vi "uc480_GetCameraList.vi"() -> ()   [LabVIEW 2011]
uses:
  C:/Program Files/Thorlabs/Scientific Imaging/DCx Camera Support/Develop/DotNet/uc480DotNet.dll
  Develop/DotNet/uc480DotNet.dll
panel:
  out "Ser.No. Camera 9":string
  out "Ser.No. Camera 8":string
  out "Ser.No. Camera 7":string
  out "Ser.No. Camera 6":string
  out "Ser.No. Camera 5":string
  out "Ser.No. Camera 4":string
  out "Ser.No. Camera 3":string
  out "Ser.No. Camera 2":string
  out "Ser.No. Camera 1":string
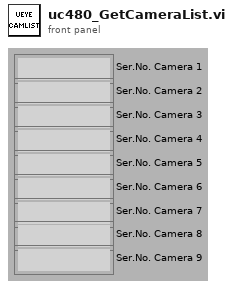
[diagram p1: front panel]
types:
  T1 = cluster{"CameraList[0]":refnum<k24>, "CameraList[1]":refnum<k24>, "CameraList[2]":refnum<k24>, "CameraList[3]":refnum<k24>, "CameraList[4]":refnum<k24>, "CameraList[5]":refnum<k24>, "CameraList[6]":refnum<k24>, "CameraList[7]":refnum<k24>, "CameraList[8]":refnum<k24>}
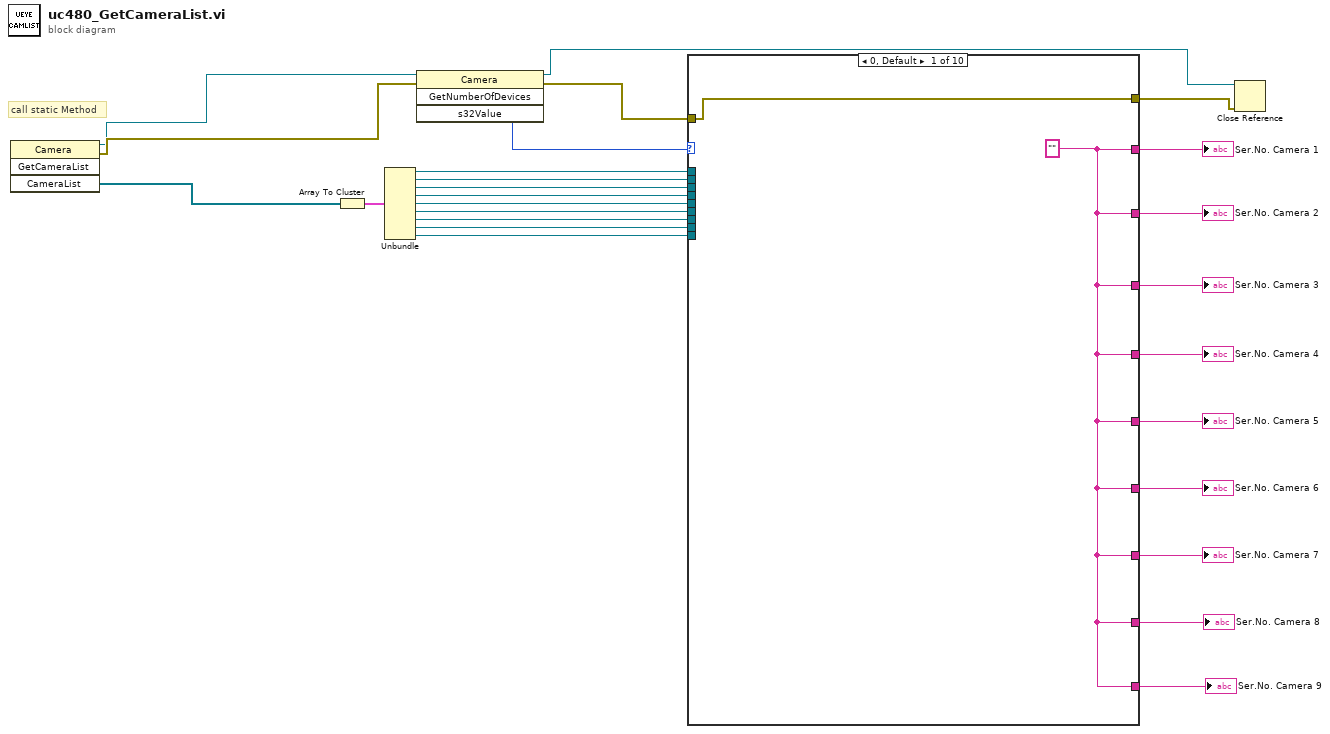
[diagram p0: block diagram]
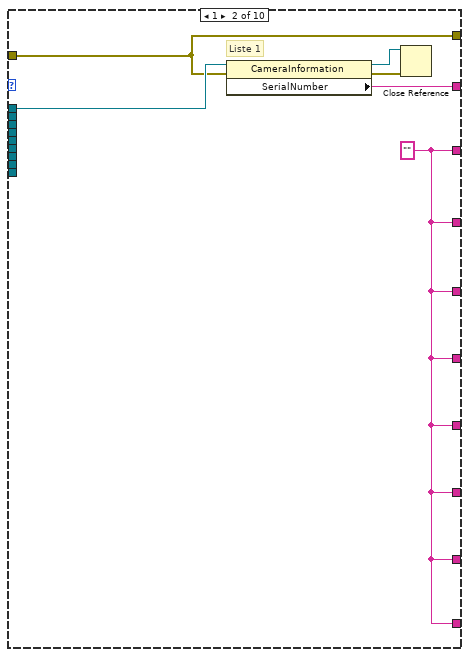
[diagram p2: hidden frame]
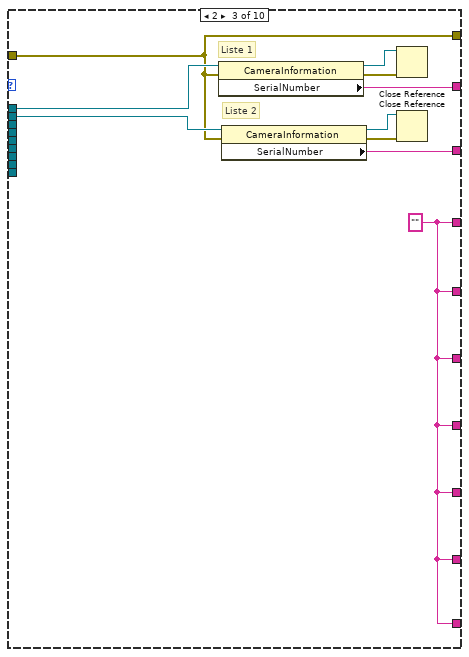
[diagram p3: hidden frame]
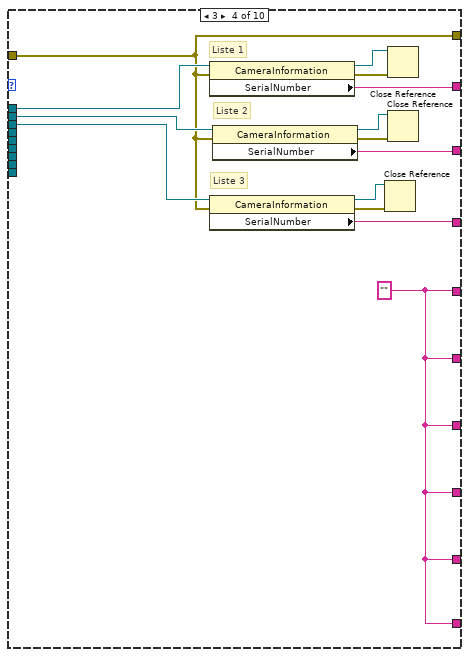
[diagram p4: hidden frame]
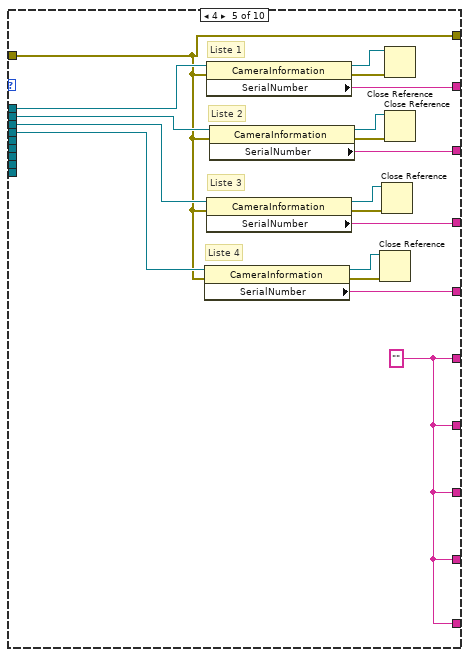
[diagram p5: hidden frame]
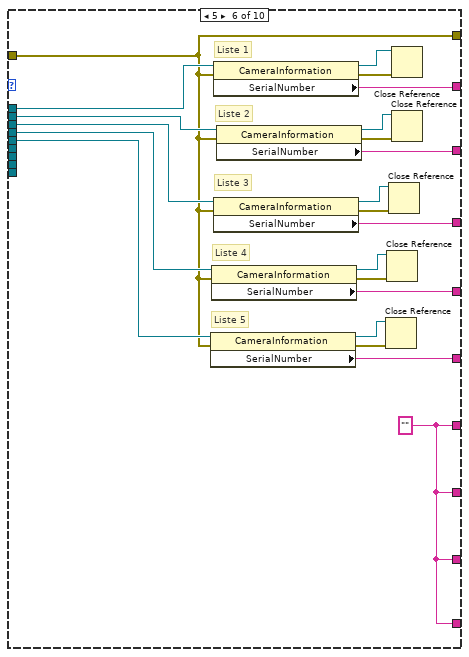
[diagram p6: hidden frame]
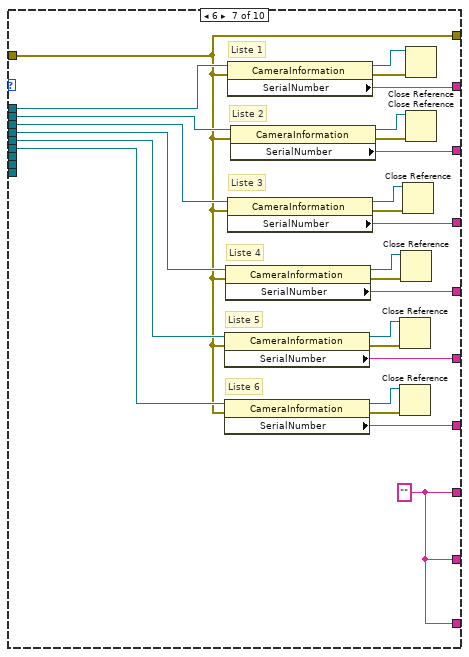
[diagram p7: hidden frame]
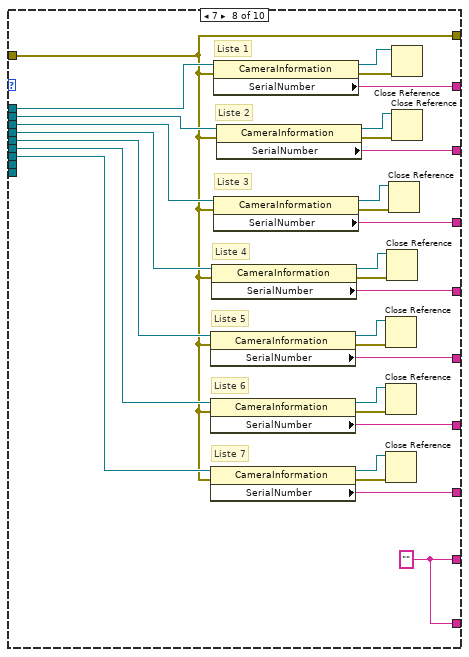
[diagram p8: hidden frame]
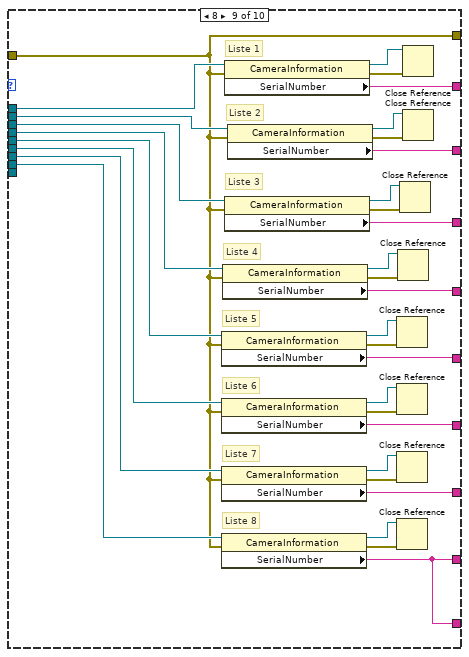
[diagram p9: hidden frame]
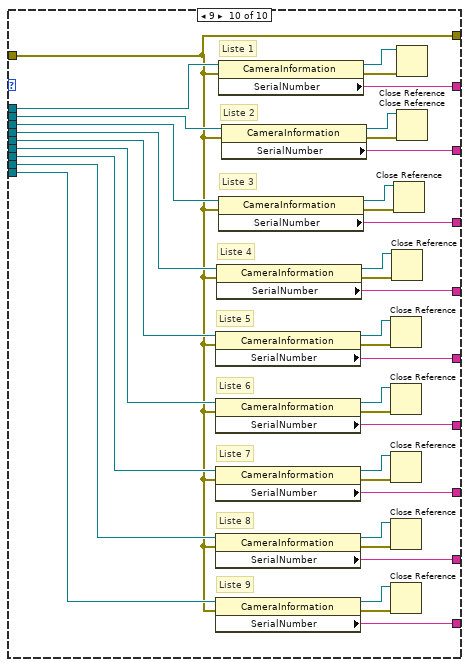
[diagram p10: hidden frame]
diagram:
  # "call static Method"
  n1 = invoke class="Camera" method="GetCameraList"() -> (reference out=w3:refnum<k24>, error out=w6:errorcluster, "CameraList"=w1:refnum<k24>[])  [unwired: 4 in, 1 out]
  n2 = Array To Cluster(array=w1) -> (cluster=w26:T1)
  n3 = Unbundle(w26) -> ("CameraList[0]"=w25:refnum<k24>, "CameraList[1]"=w22:refnum<k24>, "CameraList[2]"=w20:refnum<k24>, "CameraList[3]"=w19:refnum<k24>, "CameraList[4]"=w18:refnum<k24>, "CameraList[5]"=w17:refnum<k24>, "CameraList[6]"=w16:refnum<k24>, "CameraList[7]"=w15:refnum<k24>, "CameraList[8]"=w14:refnum<k24>)
  n4 = invoke on="Methodenknoten" class="Camera" method="GetNumberOfDevices"(reference=w3, error in=w6) -> (reference out=w2:refnum<k24>, error out=w5:errorcluster, "s32Value"=w23:i32)  [unwired: 2 in, 1 out]
  n5 = case shown="0, Default" w23 {
    tunnel: w25 -> [_ w34 w37 w49 w70 w86 w109 w136 w166 w208]
    tunnel: w5 -> [w27 w29 w35 w45 w59 w77 w99 w125 w155 w188]
    tunnel: [w28 w31 w40 w52 w67 w90 w114 w142 w173 w201] -> w24
    tunnel: w22 -> [_ _ w38 w48 w69 w85 w108 w135 w165 w207]
    tunnel: [w28 w30 w39 w51 w66 w89 w113 w141 w172 w200] -> w21
    tunnel: w20 -> [_ _ _ w47 w68 w84 w107 w134 w164 w206]
    tunnel: w19 -> [_ _ _ _ w61 w83 w106 w133 w163 w205]
    tunnel: w18 -> [_ _ _ _ _ w79 w105 w132 w162 w204]
    tunnel: w17 -> [_ _ _ _ _ _ w101 w131 w161 w203]
    tunnel: w16 -> [_ _ _ _ _ _ _ w128 w160 w202]
    tunnel: w15 -> [_ _ _ _ _ _ _ _ w157 w190]
    tunnel: w14 -> [_ _ _ _ _ _ _ _ _ w189]
    tunnel: [w28 w30 w36 w50 w65 w88 w112 w140 w171 w199] -> w13
    tunnel: [w28 w30 w36 w46 w62 w87 w111 w139 w170 w198] -> w12
    tunnel: [w28 w30 w36 w46 w60 w80 w110 w138 w169 w197] -> w11
    tunnel: [w28 w30 w36 w46 w60 w78 w102 w137 w168 w196] -> w10
    tunnel: [w28 w30 w36 w46 w60 w78 w100 w127 w167 w195] -> w9
    tunnel: [w28 w30 w36 w46 w60 w78 w100 w126 w156 w194] -> w8
    tunnel: [w28 w30 w36 w46 w60 w78 w100 w126 w156 w191] -> w7
    tunnel: [w27 w29 w35 w45 w59 w77 w99 w125 w155 w188] -> w4
    frame 0, Default {
      w28 = "" ("SerialNumber")
    }
    frame 1 {
      w30 = "" ("SerialNumber")
      # "Liste 1"
      n6 = property class="CameraInformation"(reference=w34, error in=w29) -> (reference out=w33:refnum<k24>, error out=w32:errorcluster, "SerialNumber"=w31:string)
      n7 = Close Reference(reference=w33, error in (no error)=w32) -> ()  [unwired: 1 out]
    }
    frame 2 {
      w36 = "" ("SerialNumber")
      # "Liste 2"
      # "Liste 1"
      n8 = property class="CameraInformation"(reference=w37, error in=w35) -> (reference out=w44:refnum<k24>, error out=w43:errorcluster, "SerialNumber"=w40:string)
      n9 = property class="CameraInformation"(reference=w38, error in=w35) -> (reference out=w42:refnum<k24>, error out=w41:errorcluster, "SerialNumber"=w39:string)
      n10 = Close Reference(reference=w44, error in (no error)=w43) -> ()  [unwired: 1 out]
      n11 = Close Reference(reference=w42, error in (no error)=w41) -> ()  [unwired: 1 out]
    }
    frame 3 {
      w46 = "" ("SerialNumber")
      # "Liste 3"
      # "Liste 2"
      # "Liste 1"
      n12 = property class="CameraInformation"(reference=w49, error in=w45) -> (reference out=w58:refnum<k24>, error out=w57:errorcluster, "SerialNumber"=w52:string)
      n13 = property class="CameraInformation"(reference=w47, error in=w45) -> (reference out=w54:refnum<k24>, error out=w53:errorcluster, "SerialNumber"=w50:string)
      n14 = property class="CameraInformation"(reference=w48, error in=w45) -> (reference out=w56:refnum<k24>, error out=w55:errorcluster, "SerialNumber"=w51:string)
      n15 = Close Reference(reference=w54, error in (no error)=w53) -> ()  [unwired: 1 out]
      n16 = Close Reference(reference=w58, error in (no error)=w57) -> ()  [unwired: 1 out]
      n17 = Close Reference(reference=w56, error in (no error)=w55) -> ()  [unwired: 1 out]
    }
    frame 4 {
      w60 = "" ("SerialNumber")
      # "Liste 4"
      # "Liste 3"
      # "Liste 2"
      # "Liste 1"
      n18 = property class="CameraInformation"(reference=w61, error in=w59) -> (reference out=w64:refnum<k24>, error out=w63:errorcluster, "SerialNumber"=w62:string)
      n19 = property class="CameraInformation"(reference=w70, error in=w59) -> (reference out=w76:refnum<k24>, error out=w75:errorcluster, "SerialNumber"=w67:string)
      n20 = property class="CameraInformation"(reference=w68, error in=w59) -> (reference out=w72:refnum<k24>, error out=w71:errorcluster, "SerialNumber"=w65:string)
      n21 = property class="CameraInformation"(reference=w69, error in=w59) -> (reference out=w74:refnum<k24>, error out=w73:errorcluster, "SerialNumber"=w66:string)
      n22 = Close Reference(reference=w64, error in (no error)=w63) -> ()  [unwired: 1 out]
      n23 = Close Reference(reference=w72, error in (no error)=w71) -> ()  [unwired: 1 out]
      n24 = Close Reference(reference=w76, error in (no error)=w75) -> ()  [unwired: 1 out]
      n25 = Close Reference(reference=w74, error in (no error)=w73) -> ()  [unwired: 1 out]
    }
    frame 5 {
      w78 = "" ("SerialNumber")
      # "Liste 5"
      # "Liste 4"
      # "Liste 3"
      # "Liste 2"
      # "Liste 1"
      n26 = property class="CameraInformation"(reference=w79, error in=w77) -> (reference out=w82:refnum<k24>, error out=w81:errorcluster, "SerialNumber"=w80:string)
      n27 = property class="CameraInformation"(reference=w83, error in=w77) -> (reference out=w92:refnum<k24>, error out=w91:errorcluster, "SerialNumber"=w87:string)
      n28 = property class="CameraInformation"(reference=w86, error in=w77) -> (reference out=w98:refnum<k24>, error out=w97:errorcluster, "SerialNumber"=w90:string)
      n29 = property class="CameraInformation"(reference=w84, error in=w77) -> (reference out=w94:refnum<k24>, error out=w93:errorcluster, "SerialNumber"=w88:string)
      n30 = property class="CameraInformation"(reference=w85, error in=w77) -> (reference out=w96:refnum<k24>, error out=w95:errorcluster, "SerialNumber"=w89:string)
      n31 = Close Reference(reference=w82, error in (no error)=w81) -> ()  [unwired: 1 out]
      n32 = Close Reference(reference=w92, error in (no error)=w91) -> ()  [unwired: 1 out]
      n33 = Close Reference(reference=w94, error in (no error)=w93) -> ()  [unwired: 1 out]
      n34 = Close Reference(reference=w98, error in (no error)=w97) -> ()  [unwired: 1 out]
      n35 = Close Reference(reference=w96, error in (no error)=w95) -> ()  [unwired: 1 out]
    }
    frame 6 {
      w100 = "" ("SerialNumber")
      # "Liste 6"
      # "Liste 5"
      # "Liste 4"
      # "Liste 3"
      # "Liste 2"
      # "Liste 1"
      n36 = property class="CameraInformation"(reference=w105, error in=w99) -> (reference out=w116:refnum<k24>, error out=w115:errorcluster, "SerialNumber"=w110:string)
      n37 = property class="CameraInformation"(reference=w101, error in=w99) -> (reference out=w104:refnum<k24>, error out=w103:errorcluster, "SerialNumber"=w102:string)
      n38 = property class="CameraInformation"(reference=w106, error in=w99) -> (reference out=w118:refnum<k24>, error out=w117:errorcluster, "SerialNumber"=w111:string)
      n39 = property class="CameraInformation"(reference=w109, error in=w99) -> (reference out=w124:refnum<k24>, error out=w123:errorcluster, "SerialNumber"=w114:string)
      n40 = property class="CameraInformation"(reference=w107, error in=w99) -> (reference out=w120:refnum<k24>, error out=w119:errorcluster, "SerialNumber"=w112:string)
      n41 = property class="CameraInformation"(reference=w108, error in=w99) -> (reference out=w122:refnum<k24>, error out=w121:errorcluster, "SerialNumber"=w113:string)
      n42 = Close Reference(reference=w116, error in (no error)=w115) -> ()  [unwired: 1 out]
      n43 = Close Reference(reference=w104, error in (no error)=w103) -> ()  [unwired: 1 out]
      n44 = Close Reference(reference=w118, error in (no error)=w117) -> ()  [unwired: 1 out]
      n45 = Close Reference(reference=w120, error in (no error)=w119) -> ()  [unwired: 1 out]
      n46 = Close Reference(reference=w124, error in (no error)=w123) -> ()  [unwired: 1 out]
      n47 = Close Reference(reference=w122, error in (no error)=w121) -> ()  [unwired: 1 out]
    }
    frame 7 {
      w126 = "" ("SerialNumber")
      # "Liste 7"
      # "Liste 6"
      # "Liste 5"
      # "Liste 4"
      # "Liste 3"
      # "Liste 2"
      # "Liste 1"
      n48 = property class="CameraInformation"(reference=w132, error in=w125) -> (reference out=w146:refnum<k24>, error out=w145:errorcluster, "SerialNumber"=w138:string)
      n49 = property class="CameraInformation"(reference=w131, error in=w125) -> (reference out=w144:refnum<k24>, error out=w143:errorcluster, "SerialNumber"=w137:string)
      n50 = property class="CameraInformation"(reference=w128, error in=w125) -> (reference out=w130:refnum<k24>, error out=w129:errorcluster, "SerialNumber"=w127:string)
      n51 = property class="CameraInformation"(reference=w133, error in=w125) -> (reference out=w148:refnum<k24>, error out=w147:errorcluster, "SerialNumber"=w139:string)
      n52 = property class="CameraInformation"(reference=w136, error in=w125) -> (reference out=w154:refnum<k24>, error out=w153:errorcluster, "SerialNumber"=w142:string)
      n53 = property class="CameraInformation"(reference=w134, error in=w125) -> (reference out=w150:refnum<k24>, error out=w149:errorcluster, "SerialNumber"=w140:string)
      n54 = property class="CameraInformation"(reference=w135, error in=w125) -> (reference out=w152:refnum<k24>, error out=w151:errorcluster, "SerialNumber"=w141:string)
      n55 = Close Reference(reference=w146, error in (no error)=w145) -> ()  [unwired: 1 out]
      n56 = Close Reference(reference=w144, error in (no error)=w143) -> ()  [unwired: 1 out]
      n57 = Close Reference(reference=w130, error in (no error)=w129) -> ()  [unwired: 1 out]
      n58 = Close Reference(reference=w148, error in (no error)=w147) -> ()  [unwired: 1 out]
      n59 = Close Reference(reference=w150, error in (no error)=w149) -> ()  [unwired: 1 out]
      n60 = Close Reference(reference=w154, error in (no error)=w153) -> ()  [unwired: 1 out]
      n61 = Close Reference(reference=w152, error in (no error)=w151) -> ()  [unwired: 1 out]
    }
    frame 8 {
      # "Liste 8"
      # "Liste 7"
      # "Liste 6"
      # "Liste 5"
      # "Liste 4"
      # "Liste 3"
      # "Liste 2"
      # "Liste 1"
      n62 = property class="CameraInformation"(reference=w162, error in=w155) -> (reference out=w179:refnum<k24>, error out=w178:errorcluster, "SerialNumber"=w169:string)
      n63 = property class="CameraInformation"(reference=w161, error in=w155) -> (reference out=w177:refnum<k24>, error out=w176:errorcluster, "SerialNumber"=w168:string)
      n64 = property class="CameraInformation"(reference=w160, error in=w155) -> (reference out=w175:refnum<k24>, error out=w174:errorcluster, "SerialNumber"=w167:string)
      n65 = property class="CameraInformation"(reference=w157, error in=w155) -> (reference out=w159:refnum<k24>, error out=w158:errorcluster, "SerialNumber"=w156:string)
      n66 = property class="CameraInformation"(reference=w163, error in=w155) -> (reference out=w181:refnum<k24>, error out=w180:errorcluster, "SerialNumber"=w170:string)
      n67 = property class="CameraInformation"(reference=w166, error in=w155) -> (reference out=w187:refnum<k24>, error out=w186:errorcluster, "SerialNumber"=w173:string)
      n68 = property class="CameraInformation"(reference=w164, error in=w155) -> (reference out=w183:refnum<k24>, error out=w182:errorcluster, "SerialNumber"=w171:string)
      n69 = property class="CameraInformation"(reference=w165, error in=w155) -> (reference out=w185:refnum<k24>, error out=w184:errorcluster, "SerialNumber"=w172:string)
      n70 = Close Reference(reference=w179, error in (no error)=w178) -> ()  [unwired: 1 out]
      n71 = Close Reference(reference=w177, error in (no error)=w176) -> ()  [unwired: 1 out]
      n72 = Close Reference(reference=w175, error in (no error)=w174) -> ()  [unwired: 1 out]
      n73 = Close Reference(reference=w159, error in (no error)=w158) -> ()  [unwired: 1 out]
      n74 = Close Reference(reference=w181, error in (no error)=w180) -> ()  [unwired: 1 out]
      n75 = Close Reference(reference=w183, error in (no error)=w182) -> ()  [unwired: 1 out]
      n76 = Close Reference(reference=w187, error in (no error)=w186) -> ()  [unwired: 1 out]
      n77 = Close Reference(reference=w185, error in (no error)=w184) -> ()  [unwired: 1 out]
    }
    frame 9 {
      # "Liste 9"
      # "Liste 8"
      # "Liste 7"
      # "Liste 6"
      # "Liste 5"
      # "Liste 4"
      # "Liste 3"
      # "Liste 2"
      # "Liste 1"
      n78 = property class="CameraInformation"(reference=w204, error in=w188) -> (reference out=w216:refnum<k24>, error out=w215:errorcluster, "SerialNumber"=w197:string)
      n79 = property class="CameraInformation"(reference=w203, error in=w188) -> (reference out=w214:refnum<k24>, error out=w213:errorcluster, "SerialNumber"=w196:string)
      n80 = property class="CameraInformation"(reference=w202, error in=w188) -> (reference out=w212:refnum<k24>, error out=w211:errorcluster, "SerialNumber"=w195:string)
      n81 = property class="CameraInformation"(reference=w190, error in=w188) -> (reference out=w210:refnum<k24>, error out=w209:errorcluster, "SerialNumber"=w194:string)
      n82 = property class="CameraInformation"(reference=w189, error in=w188) -> (reference out=w193:refnum<k24>, error out=w192:errorcluster, "SerialNumber"=w191:string)
      n83 = property class="CameraInformation"(reference=w205, error in=w188) -> (reference out=w218:refnum<k24>, error out=w217:errorcluster, "SerialNumber"=w198:string)
      n84 = property class="CameraInformation"(reference=w208, error in=w188) -> (reference out=w224:refnum<k24>, error out=w223:errorcluster, "SerialNumber"=w201:string)
      n85 = property class="CameraInformation"(reference=w206, error in=w188) -> (reference out=w220:refnum<k24>, error out=w219:errorcluster, "SerialNumber"=w199:string)
      n86 = property class="CameraInformation"(reference=w207, error in=w188) -> (reference out=w222:refnum<k24>, error out=w221:errorcluster, "SerialNumber"=w200:string)
      n87 = Close Reference(reference=w216, error in (no error)=w215) -> ()  [unwired: 1 out]
      n88 = Close Reference(reference=w214, error in (no error)=w213) -> ()  [unwired: 1 out]
      n89 = Close Reference(reference=w212, error in (no error)=w211) -> ()  [unwired: 1 out]
      n90 = Close Reference(reference=w210, error in (no error)=w209) -> ()  [unwired: 1 out]
      n91 = Close Reference(reference=w193, error in (no error)=w192) -> ()  [unwired: 1 out]
      n92 = Close Reference(reference=w218, error in (no error)=w217) -> ()  [unwired: 1 out]
      n93 = Close Reference(reference=w220, error in (no error)=w219) -> ()  [unwired: 1 out]
      n94 = Close Reference(reference=w224, error in (no error)=w223) -> ()  [unwired: 1 out]
      n95 = Close Reference(reference=w222, error in (no error)=w221) -> ()  [unwired: 1 out]
    }
  }
  "Ser.No. Camera 1" <- w24
  "Ser.No. Camera 2" <- w21
  "Ser.No. Camera 3" <- w13
  "Ser.No. Camera 4" <- w12
  "Ser.No. Camera 5" <- w11
  "Ser.No. Camera 6" <- w10
  "Ser.No. Camera 7" <- w9
  "Ser.No. Camera 8" <- w8
  "Ser.No. Camera 9" <- w7
  n96 = Close Reference(reference=w2, error in (no error)=w4) -> ()  [unwired: 1 out]
